vi "ConfigInstr.vi"(6 "InstrumentName":string, 7 "VisaRessIn":refnum<visa-resource-name>, 8 "error in (no error)":errorcluster caption="entrée d'erreur (pas d'erreur)", 9 "FirstClassInst":bool, 10 "Function":string, 11 "GenData In":refnum<class "Tools.lvclass"> caption="DNL_LabVIEW Object in") -> (0 "error out":errorcluster caption="sortie d'erreur", 3 "GenData Out":refnum<class "Tools.lvclass"> caption="DNL_LabVIEW Object out")   [LabVIEW 2019, in "Tools.lvclass"]
uses:
  Tools.lvclass
  C:/Programmes Labview/LabScanV1A/DevicesClass/BaseDevice/BaseDevice.lvclass
  Tools_Func.ctl
  Tools.lvclass/Tools.ctl
  BaseDevice/BaseDevice.lvclass/BaseDevice.ctl
  BaseDevice/Accessor/SetShowInstrNm.vi
  BaseDevice/Accessor/SetScanPanelPath.vi
panel:
  in  "GenData_Func":T1=enum."Courbe 2 (Arb)"
  out "VisaRessOut":refnum<visa-resource-name>
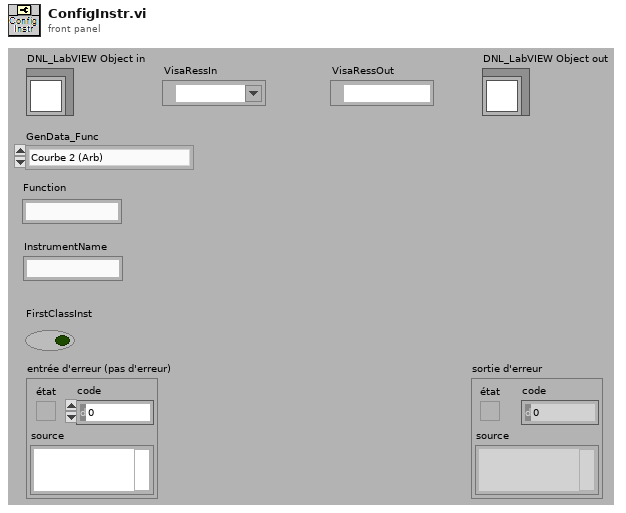
[diagram p1: front panel]
types:
  T1 = typedef "Tools.lvclass/Tools_Func.ctl" = enum16{"Courbe 1 (Arb)", "Courbe 2 (Arb)", "Courbe 3 (Arb)", "Courbe 123 (Arb,Arb,Arb)", "Scan Pos (Arb)", "Indice de Point (Points)", "AbsTime (ms)", "Minuteur (s)", "Panneaux Infos (Na)", "Délais (ms)", "RandomNum (Arb)", "Multisweep (Sw)", "ScanTime (s)"}
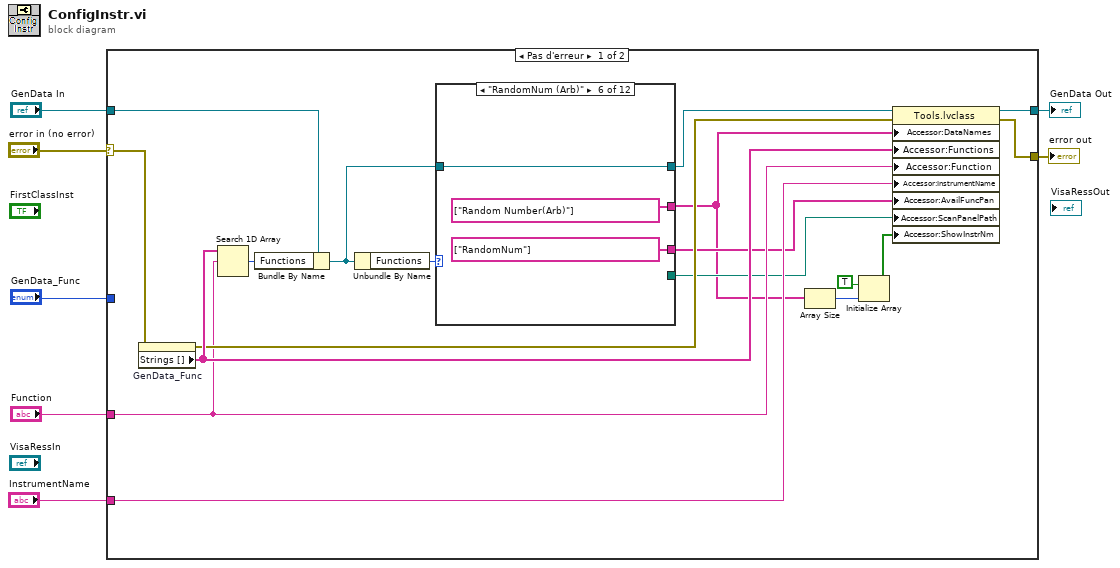
[diagram p0: block diagram]
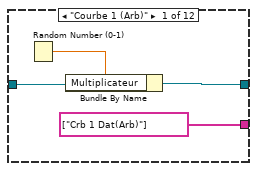
[diagram p2: hidden frame]
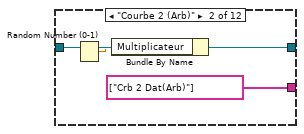
[diagram p3: hidden frame]
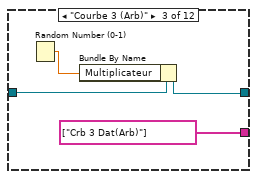
[diagram p4: hidden frame]
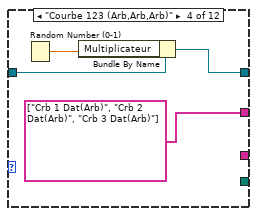
[diagram p5: hidden frame]
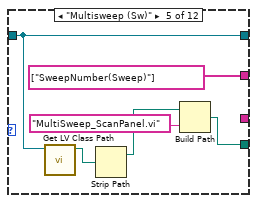
[diagram p6: hidden frame]
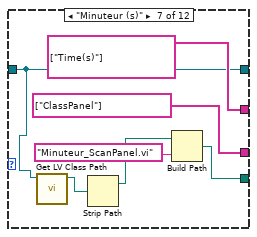
[diagram p7: hidden frame]
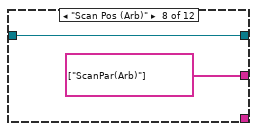
[diagram p8: hidden frame]
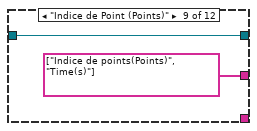
[diagram p9: hidden frame]
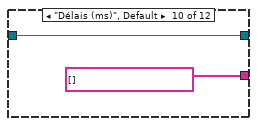
[diagram p10: hidden frame]
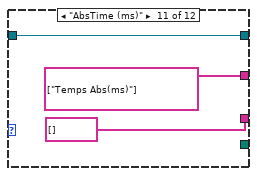
[diagram p11: hidden frame]
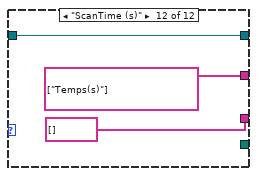
[diagram p12: hidden frame]
diagram:
  n1 = case shown="Pas d'erreur" "error in (no error)" {
    selector: "error in (no error)" -> [w19 w71]
    tunnel: [w25 w71] -> w6
    tunnel: "GenData In" -> [w20 w70]
    tunnel: [w24 w70] -> w4
    tunnel: "GenData_Func" -> [_ _]
    tunnel: "Function" -> [w15 _]
    tunnel: "InstrumentName" -> [w14 _]
    frame No Error {
      n2 = property on="GenData_Func" class="Énum (strict)"(error in=w19) -> (error out=w18:errorcluster, "Strings []"=w22:string[])  [unwired: 1 in, 1 out]
      n3 = Search 1D Array(1D array=w22, element=w15) -> (index of element=w21:i32)  [unwired: 1 in]
      n4 = Bundle By Name(cluster=w20, "Functions"=w21) -> (w17:refnum<class "Tools.lvclass">)
      n5 = Unbundle By Name(w17) -> ("Functions"=w23:T1)
      n6 = case shown="\"RandomNum (Arb)\"" w23 {
        tunnel: [string[] ["Crb 1 Dat(Arb)"] string[] ["Crb 2 Dat(Arb)"] string[] ["Crb 3 Dat(Arb)"] string[] ["Crb 1 Dat(Arb)", "Crb 2 Dat(Arb)", "Crb 3 Dat(Arb)"] string[] ["SweepNumber(Sweep)"] string[] ["Random Number(Arb)"] string[] ["Time(s)"] string[] ["ScanPar(Arb)"] string[] ["Indice de points(Points)", "Time(s)"] string[] [] string[] ["Temps Abs(ms)"] string[] ["Temps(s)"]] -> w9
        tunnel: w17 -> [w28 w32 w36 w40 w43 w49 w51 w58 w60 w62 w65 w68]
        tunnel: [w27 w31 w35 w38 w43 w49 w51 w58 w60 w62 w65 w68] -> w16
        tunnel: [_ _ _ _ _ string[] ["RandomNum"] string[] ["ClassPanel"] _ _ _ string[] [] string[] []] -> w13
        tunnel: [_ _ _ _ w42 _ w52 _ _ _ _ _] -> w12
        frame "Courbe 1 (Arb)" {
          n7 = Random Number (0-1)() -> (number: 0 to 1=w26:dbl)
          n8 = Bundle By Name(cluster=w28, "Multiplicateur"=w26) -> (w27:refnum<class "Tools.lvclass">)
        }
        frame "Courbe 2 (Arb)" {
          n9 = Random Number (0-1)() -> (number: 0 to 1=w30:dbl)
          n10 = Bundle By Name(cluster=w32, "Multiplicateur"=w30) -> (w31:refnum<class "Tools.lvclass">)
        }
        frame "Courbe 3 (Arb)" {
          n11 = Random Number (0-1)() -> (number: 0 to 1=w34:dbl)
          n12 = Bundle By Name(cluster=w36, "Multiplicateur"=w34) -> (w35:refnum<class "Tools.lvclass">)
        }
        frame "Courbe 123 (Arb,Arb,Arb)" {
          n13 = Random Number (0-1)() -> (number: 0 to 1=w39:dbl)
          n14 = Bundle By Name(cluster=w40, "Multiplicateur"=w39) -> (w38:refnum<class "Tools.lvclass">)
        }
        frame "Multisweep (Sw)" {
          n15 = call <vilib>:"Get LV Class Path.vi"("object"=w43) -> ("class path"=w46:path)  [unwired: 9 in, 1 out]
          n16 = Strip Path(path=w46) -> (stripped path=w45:path)  [unwired: 1 out]
          n17 = Build Path(base path=w45, name or relative path="MultiSweep_ScanPanel.vi") -> (appended path=w42:path)
        }
        frame "RandomNum (Arb)" {
        }
        frame "Minuteur (s)" {
          n18 = call <vilib>:"Get LV Class Path.vi"("object"=w51) -> ("class path"=w55:path)  [unwired: 9 in, 1 out]
          n19 = Strip Path(path=w55) -> (stripped path=w54:path)  [unwired: 1 out]
          n20 = Build Path(base path=w54, name or relative path="Minuteur_ScanPanel.vi") -> (appended path=w52:path)
        }
        frame "Scan Pos (Arb)" {
        }
        frame "Indice de Point (Points)" {
        }
        frame "Délais (ms)", Default {
        }
        frame "AbsTime (ms)" {
        }
        frame "ScanTime (s)" {
        }
      }
      n21 = Array Size(array=w9) -> (size(s)=w11:i32)
      n22 = Initialize Array(TRUE, w11) -> (w8:bool[])
      n23 = property class="Tools.lvclass"(reference=w16, error in=w18, "Accessor:DataNames"=w9, "Accessor:Functions"=w22, "Accessor:Function"=w15, "Accessor:InstrumentName"=w14, "Accessor:AvailFuncPan"=w13, "Accessor:ScanPanelPath"=w12, "Accessor:ShowInstrNm"=w8) -> (reference out=w24:refnum<class "Tools.lvclass">, error out=w25:errorcluster)
    }
    frame Error {
    }
  }
  "error out" <- w6
  "GenData Out" <- w4
